vi "2.vi"() -> ()   [LabVIEW 2020]
uses:
  <vilib>/Analysis/1siggen.llb/Ramp Pattern by Samples.vi
  <vilib>/Analysis/NI_AALBase.lvlib
panel:
  out "Waveform Graph":dbl[][](graph)
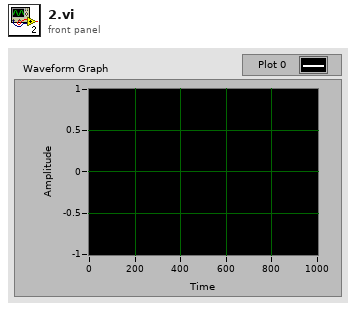
[diagram p1: front panel]
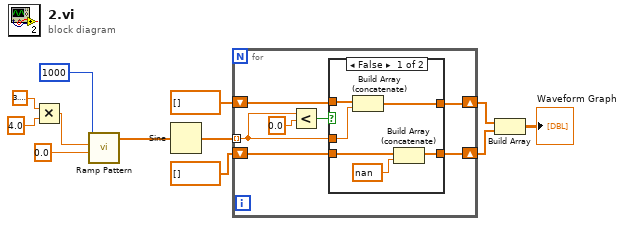
[diagram p0: block diagram]
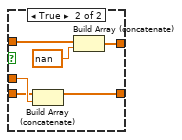
[diagram p2: hidden frame]
diagram:
  n1 = Multiply(x=3.141592653589793, y=4.0) -> (x*y=w7:dbl)
  n2 = call-poly <vilib>:"Ramp Pattern.vi"("start"=0.0, "end"=w7, "samples"=1000) -> ("Ramp Pattern"=w10:dbl[])  [unwired: 7 in, 1 out]
  n3 = Sine(x=w10) -> (sin(x)=w6:dbl[])
  n4 = for {
    tunnel: w6 -> [w13] mode=indexing
    shift-right: [w17] -> w3
    shift-left: dbl[] [] -> [w16]
    shift-right: [w15] -> w2
    shift-left: dbl[] [] -> [w14]
    n5 = Less?(x=w13, y=0.0) -> (x < y?=w18:bool)
    n6 = case shown="False" w18 {
      tunnel: [w23 w30] -> w17
      tunnel: w16 -> [w25 w29]
      tunnel: [w21 w27] -> w15
      tunnel: w14 -> [w20 w26]
      tunnel: w13 -> [w24 w28]
      frame False {
        n7 = Build Array (concatenate)(w25, w24) -> (w23:dbl[])
        n8 = Build Array (concatenate)(w20, nan) -> (w21:dbl[])
      }
      frame True {
        n9 = Build Array (concatenate)(w26, w28) -> (w27:dbl[])
        n10 = Build Array (concatenate)(w29, nan) -> (w30:dbl[])
      }
    }
  }
  n11 = Build Array(w3, w2) -> (→"Waveform Graph":dbl[][])
